vi "Clear Delete Numeric Item.vi"(5 "Target Item (0: Normal)":i32(ring) items=["Normal", "Harmonics"], 7 "Action (0: All)":i32(ring) items=["Clear All", "Clear Specific Item", "Delete Specific Item"], 8 "error in (no error)":errorcluster, 9 "Item End (255)":i32=255 min=1 max=255 step=1, 10 "Item Start (1)":i32=1 min=1 max=255 step=1, 11 "VISA resource name":refnum<visa-resource-name>) -> (0 "error out":errorcluster, 3 "VISA resource name out":refnum<visa-resource-name>)   [LabVIEW 2019, in "Yokogawa WT300 Series.lvlib"]
doc: "Clears or deletes numeric data output items."
uses:
  Yokogawa WT300 Series.lvlib
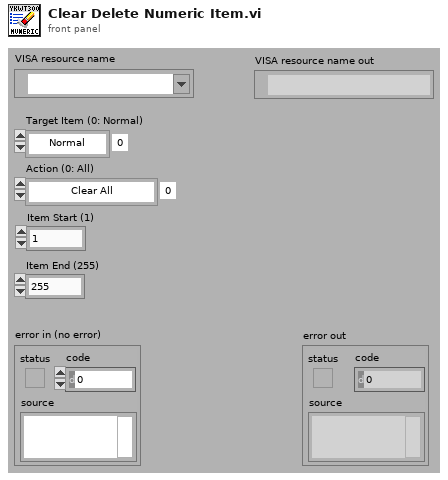
[diagram p1: front panel]
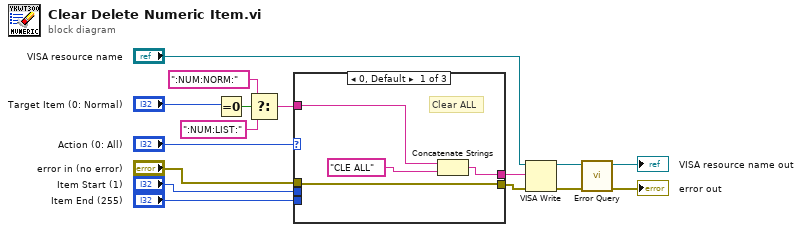
[diagram p0: block diagram]
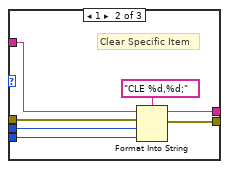
[diagram p2: hidden frame]
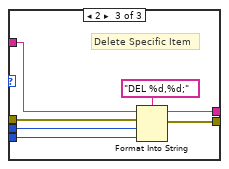
[diagram p3: hidden frame]
diagram:
  n1 = Equal To 0?(x="Target Item (0: Normal)") -> (x = 0?=w6:bool)
  n2 = Select(t=":NUM:NORM:" ("形式文字列"), s=w6, f=":NUM:LIST:" ("形式文字列")) -> (s? t:f=w2:string)
  n3 = case shown="0, Default" "Action (0: All)" {
    tunnel: "Item End (255)" -> [_ w26 w33]
    tunnel: "Item Start (1)" -> [_ w25 w32]
    tunnel: [w20 w24 w31] -> w1
    tunnel: [w19 w23 w30] -> w8
    tunnel: "error in (no error)" -> [w20 w22 w29]
    tunnel: w2 -> [w17 w21 w28]
    frame 0, Default {
      # "Clear ALL"
      n4 = Concatenate Strings(w17, "CLE ALL" ("形式文字列")) -> (w19:string)
    }
    frame 1 {
      # "Clear Specific Item"
      n5 = Format Into String(format string="CLE %d,%d;" ("形式文字列"), initial string=w21, error in=w22, w25, w26) -> (resulting string=w23:string, error out=w24:errorcluster)
    }
    frame 2 {
      # "Delete Specific Item"
      n6 = Format Into String(format string="DEL %d,%d;" ("形式文字列"), initial string=w28, error in=w29, w32, w33) -> (resulting string=w30:string, error out=w31:errorcluster)
    }
  }
  n7 = VISA Write ("VISA書き込み")(VISA resource name="VISA resource name", write buffer=w8, error in (no error)=w1) -> (VISA resource name out=w16:refnum<visa-resource-name>, error out=w15:errorcluster)  [unwired: 1 out]
  n8 = call "Error Query.vi"("error in (no error)"=w15, "VISA resource name"=w16) -> ("error out"=→"error out":errorcluster, "VISA resource name out"=→"VISA resource name out":refnum<visa-resource-name>)  [unwired: 6 in, 2 out]
